vi "RSZVB Set Status Register.vi"(5 "Enable (0)":i32, 6 "NTransition (0)":i32, 7 "PTransition (0)":i32, 8 "error in (no error)":errorcluster {"code" format="%.0x"}, 9 "Questionable Register (0: Main)":i32(ring) items=["Main", "Limit Screen A", "Limit Screen B", "Integrity", "Integrity Hardware"], 10 "Register Operation (0: Preset Registers)":i32(ring) items=["Preset Registers", "Set Questionable Register", "Set Operation Register"], 11 "VISA session":refnum<visa-resource-name>) -> (0 "error out":errorcluster {"code" format="%.0x"}, 3 "dup VISA session":refnum<visa-resource-name>)   [LabVIEW 2011]
doc: "This VI sets the Enable, NTransition, and PTransition bits of status questionable and operating registers.\n\nNote:\n\n(1) For detailed description of Status Reporting System see also operating manual.\n\nRemote-control command(s):\nSTATus:PRESet\nSTATus:QUEStionable:ENABle\nSTATus:QUEStionable:LIMit<1|2>:ENABle\nSTATus:QUEStionable:INTegrity:ENABle\nSTATus:QUEStionable:INTegrity:HARDware:ENABle\nSTATus:QUEStionable:PTRansition\nSTATus:QUEStionable:LIMit<1|2>:PTRansition\nSTATus:QUEStionable:INTegrity:PTRansition\nSTATus:QUEStionable:INTegrity:HARDware:PTRansition\nSTATus:QUEStionable:NTRansition\nSTATus:QUEStionable:LIMit<1|2>:NTRansition\nSTATus:QUEStionable:INTegrity:NTRansition\nSTATus:QUEStionable:INTegrity:HARDware:NTRansition"
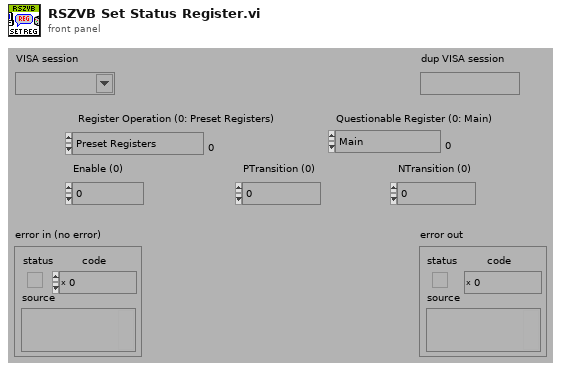
[diagram p1: front panel]
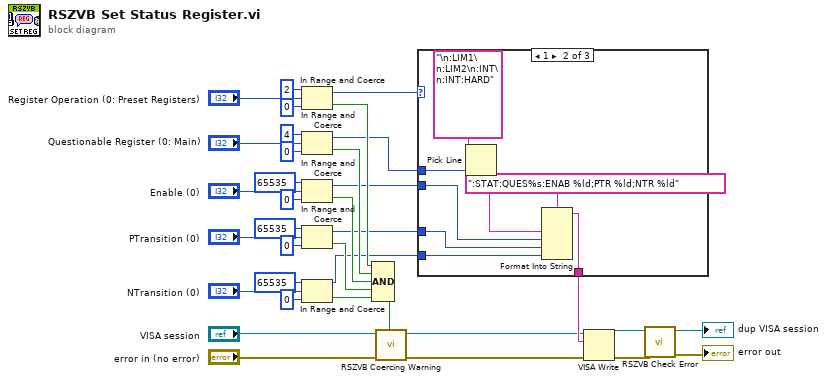
[diagram p0: block diagram]
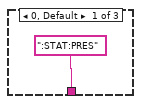
[diagram p2: hidden frame]
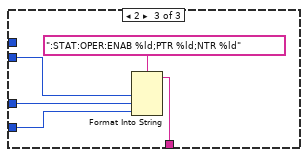
[diagram p3: hidden frame]
diagram:
  n1 = In Range and Coerce(upper limit=2, x="Register Operation (0: Preset Registers)", lower limit=0) -> (coerced(x)=w19:i32, In Range?=w24:bool)
  n2 = In Range and Coerce(upper limit=4, x="Questionable Register (0: Main)", lower limit=0) -> (coerced(x)=w15:i32, In Range?=w23:bool)
  n3 = In Range and Coerce(upper limit=65535, x="Enable (0)", lower limit=0) -> (coerced(x)=w18:i32, In Range?=w22:bool)
  n4 = In Range and Coerce(upper limit=65535, x="PTransition (0)", lower limit=0) -> (coerced(x)=w17:i32, In Range?=w21:bool)
  n5 = In Range and Coerce(upper limit=65535, x="NTransition (0)", lower limit=0) -> (coerced(x)=w16:i32, In Range?=w20:bool)
  n6 = Compound Arithmetic op=AND(w24, w23, w22, w21, w20) -> (w2:bool)
  n7 = call "RSZVB Coercing Warning.vi"("In Range?"=w2, "error in (no error)"="error in (no error)", "VISA session"="VISA session") -> ("error out"=w8:errorcluster, "dup VISA session"=w9:refnum<visa-resource-name>)  [unwired: 7 in]
  n8 = case shown="1" w19 {
    tunnel: [":STAT:PRES" w44 w48] -> w35
    tunnel: w18 -> [_ w43 w47]
    tunnel: w17 -> [_ w42 w46]
    tunnel: w16 -> [_ w41 w45]
    tunnel: w15 -> [_ w38 _]
    frame 0, Default {
    }
    frame 1 {
      n9 = Pick Line(multi-line string="\n:LIM1\n:LIM2\n:INT\n:INT:HARD", line index=w38) -> (output string=w39:string)  [unwired: 1 in]
      n10 = Format Into String(format string=":STAT:QUES%s:ENAB %ld;PTR %ld;NTR %ld", w39, w43, w42, w41) -> (resulting string=w44:string)  [unwired: 2 in, 1 out]
    }
    frame 2 {
      n11 = Format Into String(format string=":STAT:OPER:ENAB %ld;PTR %ld;NTR %ld", w47, w46, w45) -> (resulting string=w48:string)  [unwired: 2 in, 1 out]
    }
  }
  n12 = VISA Write(VISA resource name=w9, write buffer=w35, error in (no error)=w8) -> (VISA resource name out=w11:refnum<visa-resource-name>, error out=w14:errorcluster)  [unwired: 1 out]
  n13 = call "RSZVB Check Error.vi"("error in (no error)"=w14, "VISA session"=w11) -> ("error out"=→"error out":errorcluster, "dup VISA session"=→"dup VISA session":refnum<visa-resource-name>)  [unwired: 8 in]
